vi "Cryotel Read Status.vi"(8 "error in":errorcluster, 10 "Number of reads":i32=1, 11 "VISA Resource (write)":refnum<visa-resource-name>="COM1") -> (0 "error out":errorcluster, 2 "Data":dbl[](array[numeric]), 3 "Raw String Responses":string[](array[string]))   [LabVIEW 2024]
uses:
  <vilib>/Analysis/baseanly.llb/Mean (DBL).vi
  <vilib>/Analysis/NI_AALBase.lvlib
panel:
  out "Array":string[](array[string])
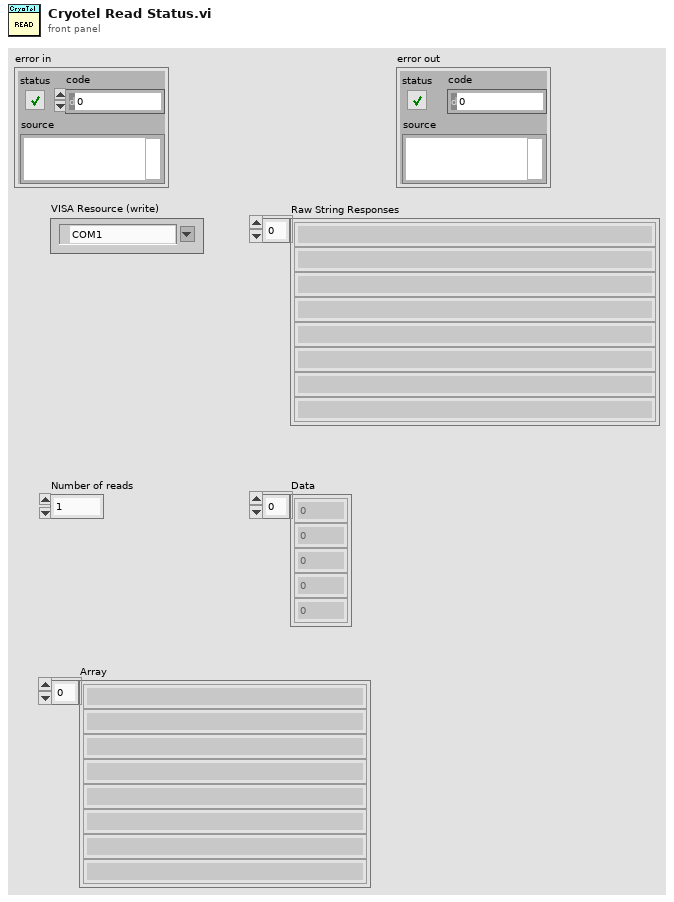
[diagram p1: front panel]
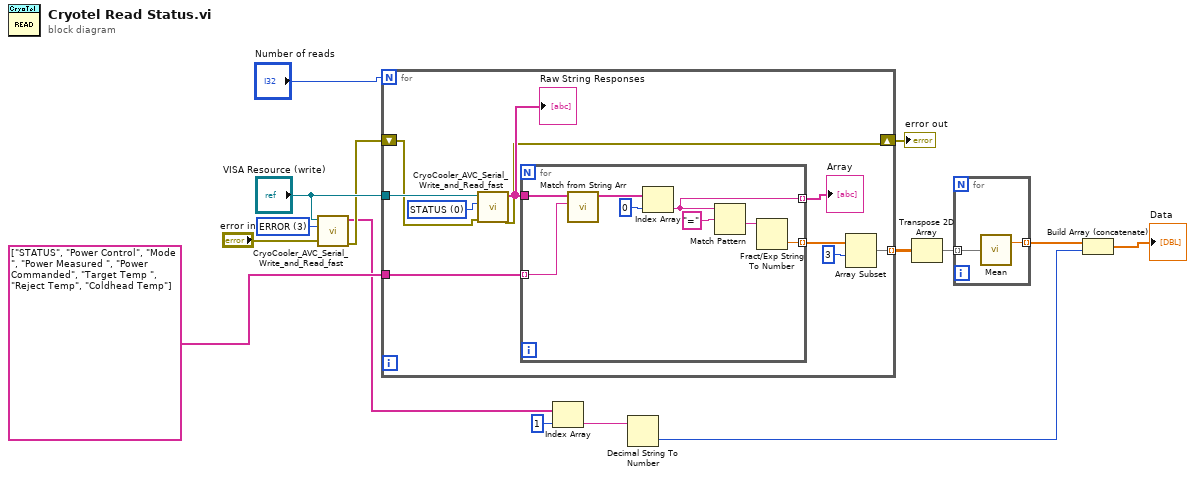
[diagram p0: block diagram]
diagram:
  w6 = u16 3 items=["STATUS", "COOLER", "E", "ERROR", "KD", "KI", "KP", "LOGIN", "LOGOUT", "MODE", "P", "PWOUT", "SENSOR", "TC", "TEMP RJ", "TTARGET", "VERSION"] ("Command")
  n1 = call "CryoCooler_AVC_Serial_Write_and_Read_fast.vi"("error in (no error)"="error in", "Command"=w6, "VISA Resource (write)"="VISA Resource (write)") -> ("error out"=w7:errorcluster, "read string array"=w5:string[])  [unwired: 6 in, 1 out]
  n2 = for {
    N: "Number of reads" -> [_]
    tunnel: [w22] -> w12 mode=indexing
    tunnel: string[] ["STATUS", "Power Control", "Mode  ", "Power Measured ", "Power Commanded", "Target Temp ", "Reject Temp", "Coldhead Temp"] -> [w20]
    tunnel: "VISA Resource (write)" -> [w19]
    shift-right: [w17] -> w10
    shift-left: w7 -> [w16]
    w18 = u16 0 items=["STATUS", "COOLER", "E", "ERROR", "KD", "KI", "KP", "LOGIN", "LOGOUT", "MODE", "P", "PWOUT", "SENSOR", "TC", "TEMP RJ", "TTARGET", "VERSION"] ("Command")
    n3 = call "CryoCooler_AVC_Serial_Write_and_Read_fast.vi"("error in (no error)"=w16, "Command"=w18, "VISA Resource (write)"=w19) -> ("error out"=w17:errorcluster, "read string array"=w21:string[])  [unwired: 6 in, 1 out]
    "Raw String Responses" <- w21
    n4 = for {
      tunnel: w21 -> [w33]
      tunnel: [w29] -> w25 mode=indexing
      tunnel: [w30] -> w23 mode=indexing
      tunnel: w20 -> [w26] mode=indexing
      n5 = call "Match from String Arr.vi"("String to match"=w26, "String Array In"=w33) -> ("String Array Matched"=w32:string[])  [unwired: 6 in, 3 out]
      n6 = Index Array(array=w32, index=0) -> (element=w29:string)
      n7 = Match Pattern(string=w29, regular expression="=") -> (after substring=w27:string)  [unwired: 1 in, 3 out]
      n8 = Fract/Exp String To Number(string=w27) -> (number=w30:dbl)  [unwired: 3 in, 1 out]
    }
    "Array" <- w25
    n9 = Array Subset(array=w23, index=3) -> (w22:dbl[])  [unwired: 1 in]
  }
  "error out" <- w10
  n10 = Index Array(array=w5, index=1) -> (element=w2:string)
  n11 = Decimal String To Number(string=w2) -> (number=w1:i32)  [unwired: 2 in, 1 out]
  n12 = Transpose 2D Array(2D array=w12) -> (transposed array=w13:dbl[][])
  n13 = for {
    tunnel: w13 -> [w35] mode=indexing
    tunnel: [w34] -> w11 mode=indexing
    n14 = call-poly <vilib>:"Mean.vi"("X"=w35) -> ("mean"=w34:dbl)  [unwired: 1 out]
  }
  n15 = Build Array (concatenate)(w11, w1) -> (→"Data":dbl[])
